vi "Write Field Size.vi"(8 "error in (no error)":errorcluster, 10 "Field Size 2":T1, 11 "Vision in":refnum<class "Vision.lvclass">) -> (0 "error out":errorcluster, 3 "Vision out":refnum<class "Vision.lvclass">)   [LabVIEW 2022 SP3, in "Vision.lvclass"]
uses:
  Vision.lvclass
  Old vision/SSL Detection Frame Simple Estimator Cameras VelCmd Folder/Core/Field Size.ctl
  Vision.lvclass/Vision.ctl
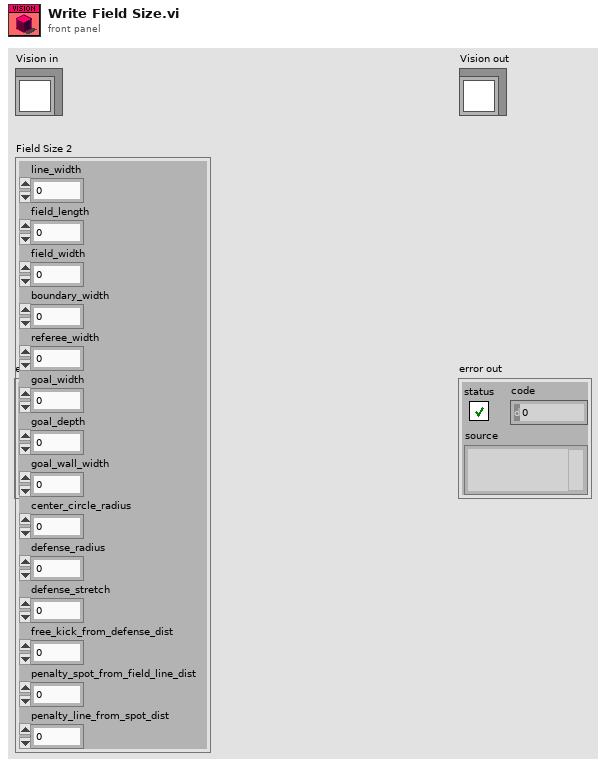
[diagram p1: front panel]
types:
  T1 = typedef "Field Size.ctl" = cluster{"line_width":u32, "field_length":u32, "field_width":u32, "boundary_width":u32, "referee_width":u32, "goal_width":u32, "goal_depth":u32, "goal_wall_width":u32, "center_circle_radius":u32, "defense_radius":u32, "defense_stretch":u32, "free_kick_from_defense_dist":u32, "penalty_spot_from_field_line_dist":u32, "penalty_line_from_spot_dist":u32}
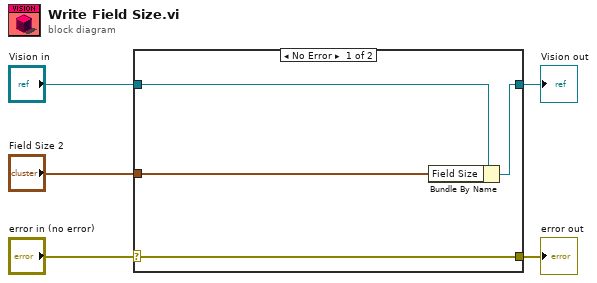
[diagram p0: block diagram]
diagram:
  n1 = case shown="No Error" "error in (no error)" {
    selector: "error in (no error)" -> [w9 w10]
    tunnel: [w9 w10] -> w4
    tunnel: [w7 w11] -> w2
    tunnel: "Vision in" -> [w8 w11]
    tunnel: "Field Size 2" -> [w6 _]
    frame No Error {
      n2 = Bundle By Name(cluster=w8, "Field Size"=w6) -> (w7:refnum<class "Vision.lvclass">)
    }
    frame Error {
    }
  }
  "error out" <- w4
  "Vision out" <- w2
